vi "Teleop - Drive Control.vi"(10 "Joystick 0 Buttons":bool[](array[boolean]), 11 "Joystick 0 Axes":dbl[](array[numeric])) -> ()   [LabVIEW 2017]
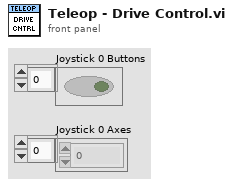
[diagram p1: front panel]
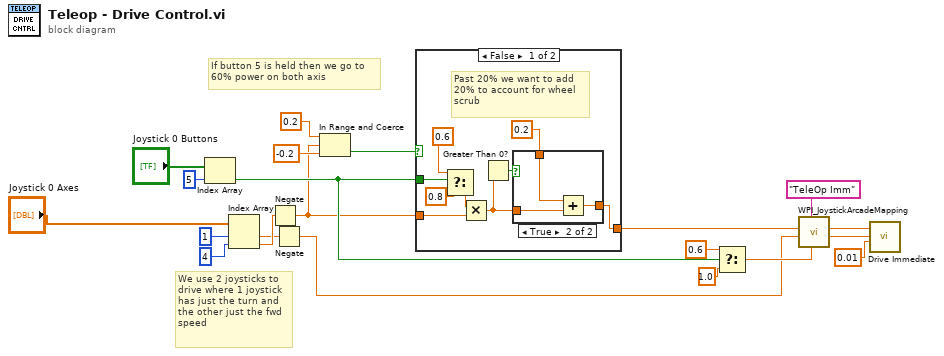
[diagram p0: block diagram]
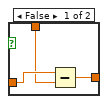
[diagram p2: hidden frame]
diagram:
  # "We use 2 joysticks to\ndrive where 1 joystick\nhas just the turn and\nthe other just the fwd\nspeed"
  # "If button 5 is held then we go to\n60% power on both axis"
  n1 = Index Array(array="Joystick 0 Buttons", index=5) -> (element=w16:bool)
  n2 = Index Array(array="Joystick 0 Axes", index #1=1 ("index"), index #2=4 ("index")) -> (element #1=w2:dbl, element #2=w4:dbl)
  n3 = Negate(x=w4) -> (-x=w12:dbl)
  n4 = Negate(x=w2) -> (-x=w3:dbl)
  n5 = In Range and Coerce(upper limit=0.2, x=w12, lower limit=-0.2) -> (In Range?=w11:bool)  [unwired: 1 out]
  n6 = case shown="False" w11 {
    tunnel: w12 -> [w30 w37]
    tunnel: w16 -> [w29 _]
    tunnel: [w23 w37] -> w5
    frame False {
      # "Past 20% we want to add\n20% to account for wheel\nscrub"
      n7 = Select(t=0.6, s=w29, f=0.8) -> (s? t:f=w26:dbl)
      n8 = Multiply(x=w26, y=w30) -> (x*y=w25:dbl)
      n9 = Greater Than 0?(x=w25) -> (x > 0?=w24:bool)
      n10 = case shown="True" w24 {
        tunnel: w25 -> [w32 w36]
        tunnel: [w33 w35] -> w23
        tunnel: 0.2 ("x") -> [w31 w34]
        frame False {
          n11 = Subtract(x=w32, y=w31) -> (x-y=w33:dbl)
        }
        frame True {
          n12 = Add(x=w34, y=w36) -> (x+y=w35:dbl)
        }
      }
    }
    frame True {
      # "Stick is near 0 so just\nuse the raw output\nfor small turns"
    }
  }
  n13 = Select(t=0.6, s=w16, f=1.0) -> (s? t:f=w19:dbl)
  n14 = call <vilib>:"WPI_JoystickArcadeMapping.vi"("Max Output"=w19, "Y axis value"=w3, "X axis value"=w5) -> ("Right Motor Value"=w8:dbl, "Left Motor Value"=w7:dbl)  [unwired: 7 in]
  n15 = call "Drive Immediate.vi"("Description"="TeleOp Imm", "Deadband Value"=0.01, "Right Setpoint"=w8, "Left Setpoint"=w7) -> ()  [unwired: 7 in, 1 out]
